vi "Load array.vi"(8 "Error In":errorcluster, 9 "Amplitude data":T1 {"Channel 31" min=0.0 max=204.7875 step=0.012500000186264515 format="%#_g V"; "Channel 30" min=0.0 max=204.7875 step=0.012500000186264515 format="%#_g V"; "Channel 29" min=0.0 max=204.7875 step=0.012500000186264515 format="%#_g V"; "Channel 28" min=0.0 max=204.7875 step=0.012500000186264515 format="%#_g V"; "Channel 27" min=0.0 max=204.7875 step=0.012500000186264515 format="%#_g V"; "Channel 26" min=0.0 max=204.7875 step=0.012500000186264515 format="%#_g V"; "Channel 25" min=0.0 max=204.7875 step=0.012500000186264515 format="%#_g V"; "Channel 24" min=0.0 max=204.7875 step=0.012500000186264515 format="%#_g V"; "Channel 23" min=0.0 max=204.7875 step=0.012500000186264515 format="%#_g V"; "Channel 22" min=0.0 max=204.7875 step=0.012500000186264515 format="%#_g V"; "Channel 21" min=0.0 max=204.7875 step=0.012500000186264515 format="%#_g V"; "Channel 20" min=0.0 max=204.7875 step=0.012500000186264515 format="%#_g V"; "Channel 19" min=0.0 max=204.7875 step=0.012500000186264515 format="%#_g V"; "Channel 18" min=0.0 max=204.7875 step=0.012500000186264515 format="%#_g V"; "Channel 17" min=0.0 max=204.7875 step=0.012500000186264515 format="%#_g V"; "Channel 16" min=0.0 max=204.7875 step=0.012500000186264515 format="%#_g V"; "Channel 15" min=0.0 max=204.7875 step=0.012500000186264515 format="%#_g V"; "Channel 14" min=0.0 max=204.7875 step=0.012500000186264515 format="%#_g V"; "Channel 13" min=0.0 max=204.7875 step=0.012500000186264515 format="%#_g V"; "Channel 12" min=0.0 max=204.7875 step=0.012500000186264515 format="%#_g V"; "Channel 11" min=0.0 max=204.7875 step=0.012500000186264515 format="%#_g V"; "Channel 10" min=0.0 max=204.7875 step=0.012500000186264515 format="%#_g V"; "Channel 9" min=0.0 max=204.7875 step=0.012500000186264515 format="%#_g V"; "Channel 8" min=0.0 max=204.7875 step=0.012500000186264515 format="%#_g V"; "Channel 7" min=0.0 max=204.7875 step=0.012500000186264515 format="%#_g V"; "Channel 6" min=0.0 max=204.7875 step=0.012500000186264515 format="%#_g V"; "Channel 5" min=0.0 max=204.7875 step=0.012500000186264515 format="%#_g V"; "Channel 4" min=0.0 max=204.7875 step=0.012500000186264515 format="%#_g V"; "Channel 3" min=0.0 max=204.7875 step=0.012500000186264515 format="%#_g V"; "Channel 2" min=0.0 max=204.7875 step=0.012500000186264515 format="%#_g V"; "Channel 1" min=0.0 max=204.7875 step=0.012500000186264515 format="%#_g V"}, 10 "Frequency":dbl=0.5 min=0.5 max=500.0 step=0.5 format="%#_g Hz", 11 "Arduino port in":refnum<visa-resource-name>) -> (0 "Error Out":errorcluster, 3 "Arduino port out":refnum<visa-resource-name>)   [LabVIEW 2016]
uses:
  Typedef/AD5535 - Command.ctl
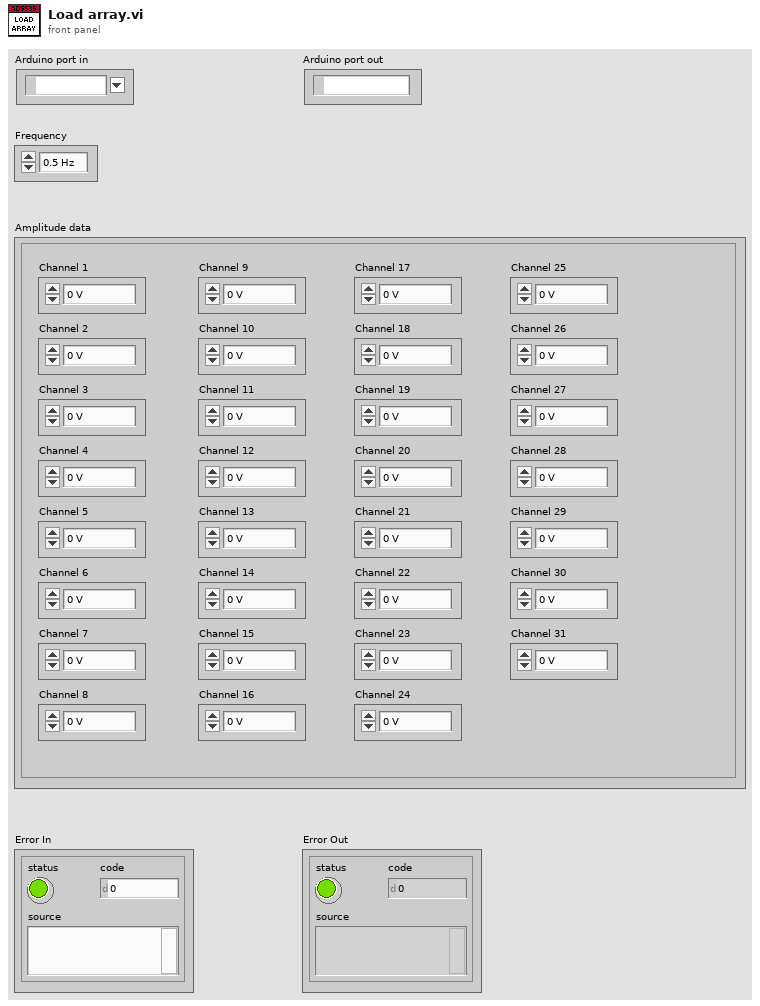
[diagram p1: front panel]
types:
  T1 = cluster{"Channel 1":dbl, "Channel 2":dbl, "Channel 3":dbl, "Channel 4":dbl, "Channel 5":dbl, "Channel 6":dbl, "Channel 7":dbl, "Channel 8":dbl, "Channel 9":dbl, "Channel 10":dbl, "Channel 11":dbl, "Channel 12":dbl, "Channel 13":dbl, "Channel 14":dbl, "Channel 15":dbl, "Channel 16":dbl, "Channel 17":dbl, "Channel 18":dbl, "Channel 19":dbl, "Channel 20":dbl, "Channel 21":dbl, "Channel 22":dbl, "Channel 23":dbl, "Channel 24":dbl, "Channel 25":dbl, "Channel 26":dbl, "Channel 27":dbl, "Channel 28":dbl, "Channel 29":dbl, "Channel 30":dbl, "Channel 31":dbl}
  T2 = typedef "AD5535 - Command.ctl" = enum16{"None", "Start", "Stop", "Load Array", "Update channel", "Update frequency", "Prova"}
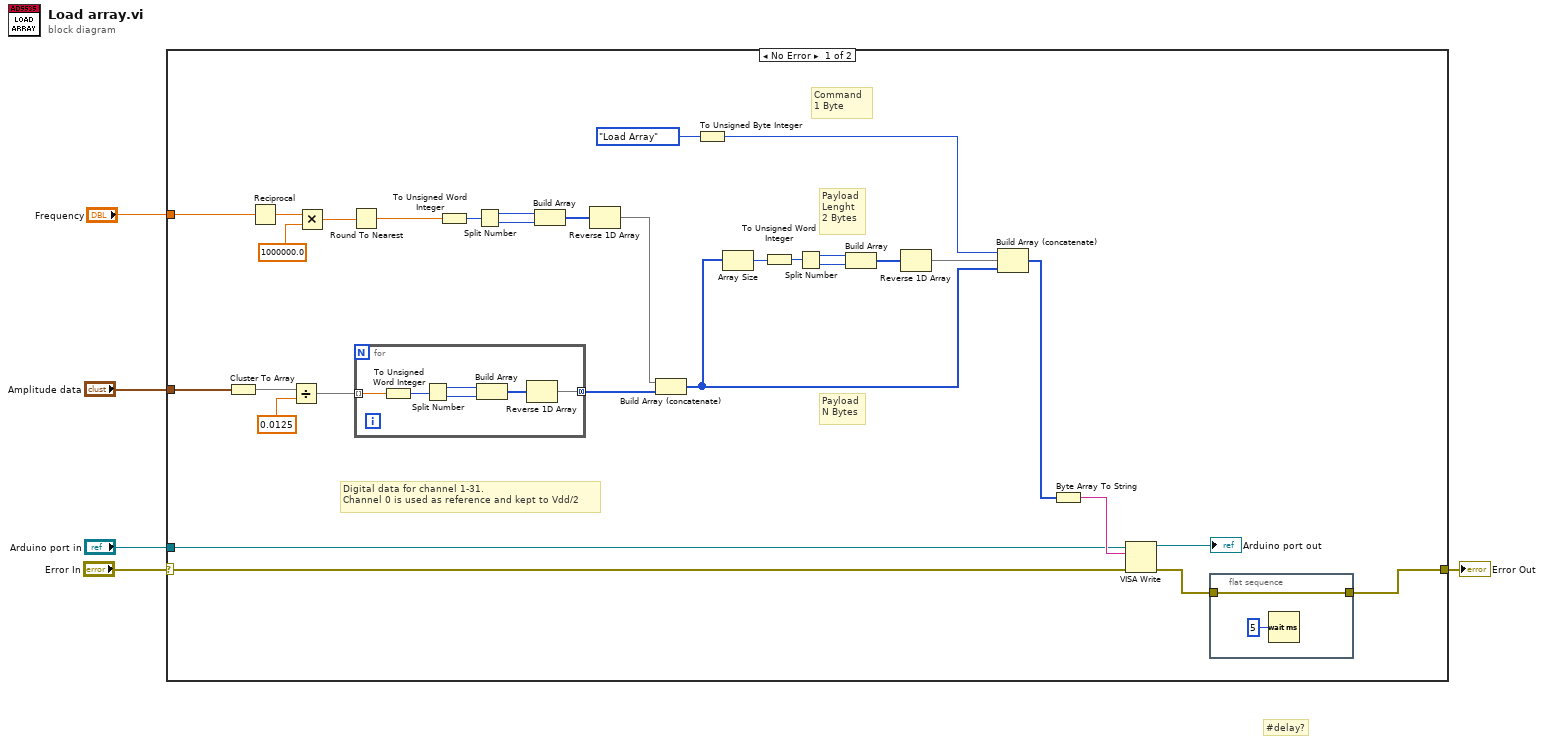
[diagram p0: block diagram]
diagram:
  # "#delay?"
  n1 = case shown="No Error" "Error In" {
    selector: "Error In" -> [w36 w45]
    tunnel: [w6 w45] -> w4
    tunnel: "Frequency" -> [w26 _]
    tunnel: "Arduino port in" -> [w33 _]
    tunnel: "Amplitude data" -> [w25 _]
    frame No Error {
      # "Payload\nLenght\n2 Bytes"
      # "Digital data for channel 1-31.\nChannel 0 is used as reference and kept to Vdd/2"
      # "Payload\nN Bytes"
      # "Command\n1 Byte"
      n2 = Cluster To Array(cluster=w25) -> (array=w24:dbl[])
      n3 = Reciprocal(x=w26) -> (1/x=w32:dbl)
      n4 = Divide(x=w24, y=0.0125) -> (x/y=w22:dbl[])
      n5 = Multiply(x=w32, y=1000000.0) -> (x*y=w30:dbl)
      n6 = Round To Nearest(number=w30) -> (nearest integer value=w28:dbl)
      n7 = for {
        tunnel: w22 -> [w44] mode=indexing
        tunnel: [w39] -> w21 mode=concatenating
        n8 = To Unsigned Word Integer(number=w44) -> (unsigned 16bit integer=w43:u16)
        n9 = Split Number(x=w43) -> (hi(x)=w42:u8, lo(x)=w41:u8)
        n10 = Build Array(w42, w41) -> (w40:u8[])
        n11 = Reverse 1D Array(array=w40) -> (reversed array=w39:u8[])
      }
      n12 = To Unsigned Word Integer(number=w28) -> (unsigned 16bit integer=w27:u16)
      n13 = Split Number(x=w27) -> (hi(x)=w13:u8, lo(x)=w12:u8)
      n14 = Build Array(w13, w12) -> (w11:u8[])
      n15 = Reverse 1D Array(array=w11) -> (reversed array=w10:u8[])
      n16 = Build Array (concatenate)(w10, w21) -> (w19:u8[])
      n17 = To Unsigned Byte Integer(number=AD5535_-_Command."Load Array" ("AD5535 - Command")) -> (unsigned 8bit integer=w20:u8)
      n18 = Array Size(array=w19) -> (size(s)=w17:i32)
      n19 = To Unsigned Word Integer(number=w17) -> (unsigned 16bit integer=w16:u16)
      n20 = Split Number(x=w16) -> (hi(x)=w15:u8, lo(x)=w14:u8)
      n21 = Build Array(w15, w14) -> (w9:u8[])
      n22 = Reverse 1D Array(array=w9) -> (reversed array=w8:u8[])
      n23 = Build Array (concatenate)(w20, w8, w19) -> (w18:u8[])
      n24 = Byte Array To String(unsigned byte array=w18) -> (string=w34:string)
      n25 = VISA Write(VISA resource name=w33, write buffer=w34, error in (no error)=w36) -> (VISA resource name out=→"Arduino port out":refnum<visa-resource-name>, error out=w7:errorcluster)  [unwired: 1 out]
      n26 = flat-sequence {
        tunnel: w7 -> [w37]
        tunnel: [w37] -> w6
        frame #0 {
          n27 = Wait (ms)(milliseconds to wait=u32 5) -> ()  [unwired: 1 out]
        }
      }
    }
    frame Error {
    }
  }
  "Error Out" <- w4
